vi "_word.table.Headers.vi"(7 "word.application":refnum<k7>, 8 "error in (no error)":errorcluster, 11 "table in":refnum<k7>) -> (0 "error out":errorcluster, 2 "table row contents":string[](array[string]), 3 "table out":refnum<k7>)   [LabVIEW 2018, in "WordReportGeneration.lvlib"]
uses:
  WordReportGeneration.lvlib
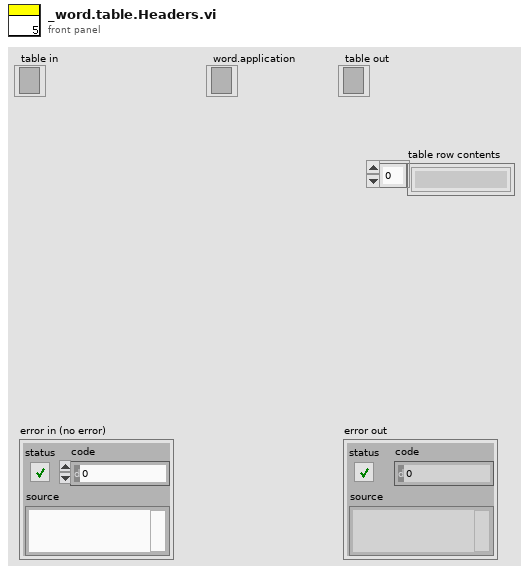
[diagram p1: front panel]
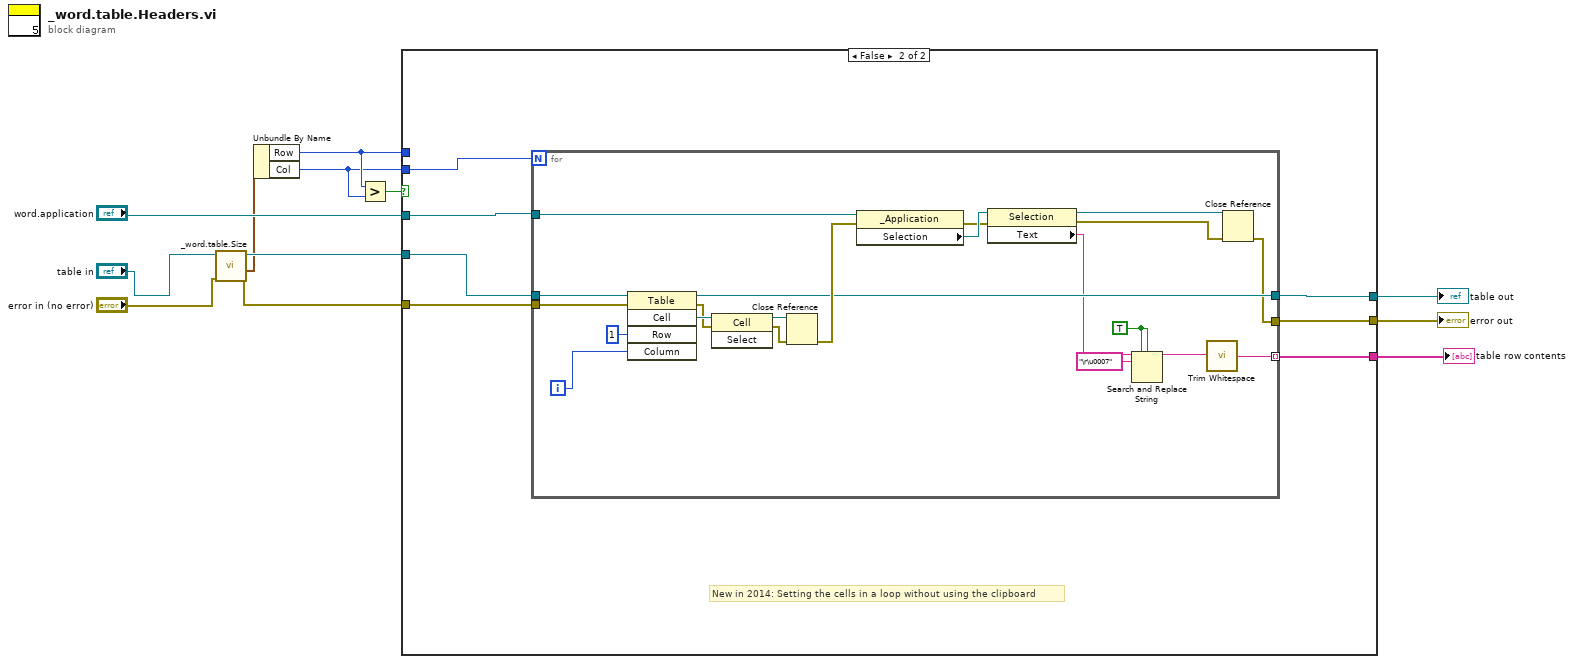
[diagram p0: block diagram]
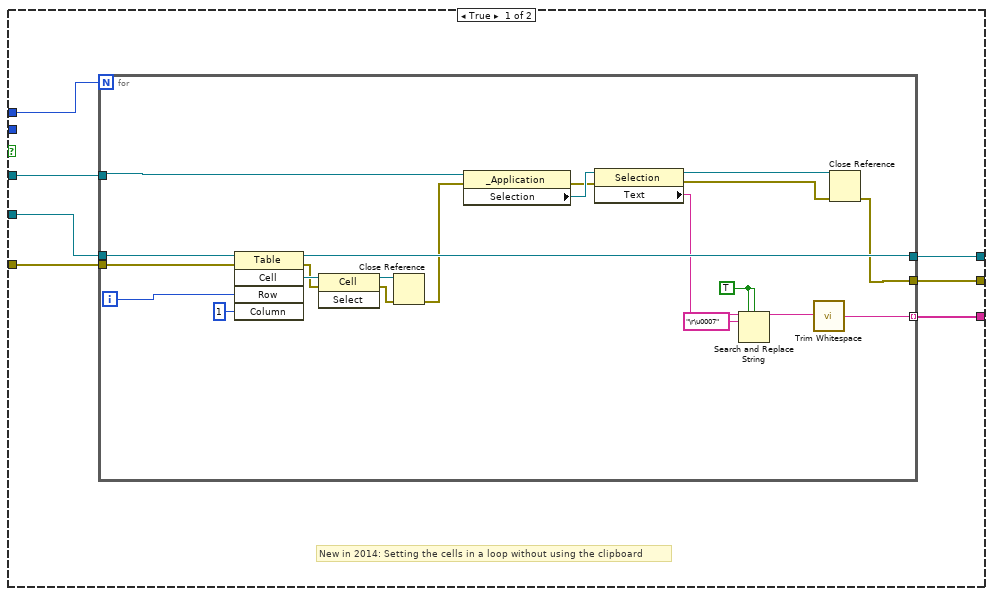
[diagram p2: hidden frame]
diagram:
  n1 = call "_word.table.Size.vi"("error in (no error)"="error in (no error)", "table Refnum in"="table in") -> ("error out"=w6:errorcluster, "Cluster"=w5:cluster{"Row":i32, "Col":i32}, "table Refnum out"=w8:refnum<k7>)  [unwired: 7 in]
  n2 = Unbundle By Name(w5) -> ("Row"=w4:i32, "Col"=w3:i32)
  n3 = Greater?(x=w4, y=w3) -> (0:w2:bool)
  n4 = case shown="False" w2 {
    tunnel: [w19 w47] -> w12
    tunnel: [w18 w46] -> w11
    tunnel: "word.application" -> [w17 w45]
    tunnel: w8 -> [w16 w44]
    tunnel: w6 -> [w15 w43]
    tunnel: [w13 w42] -> w1
    tunnel: w4 -> [w14 _]
    tunnel: w3 -> [_ w41]
    frame True {
      # "New in 2014: Setting the cells in a loop without using the clipboard"
      n5 = for {
        N: w14 -> [_]
        tunnel: [w40] -> w18
        tunnel: [w39] -> w19
        tunnel: w15 -> [w37]
        tunnel: w17 -> [w36]
        tunnel: w16 -> [w35]
        tunnel: [w34] -> w13 mode=indexing
        i -> [w38]
        w22 = TRUE ("ignore case? (F)")
        n6 = invoke class="Table" method="Cell"(reference=w35, error in=w37, "Row"=w38, "Column"=1) -> (reference out=w40:refnum<k7>, error out=w32:errorcluster, "Cell"=w33:refnum<k7>)  [unwired: 1 in, 2 out]
        n7 = invoke class="Cell" method="Select"(reference=w33, error in=w32) -> (reference out=w29:refnum<k7>, error out=w31:errorcluster)  [unwired: 1 in, 1 out]
        n8 = Close Reference(reference=w29, error in (no error)=w31) -> (error out=w30:errorcluster)
        n9 = property class="_Application"(reference=w36, error in=w30) -> (error out=w25:errorcluster, "Selection"=w26:refnum<k7>)  [unwired: 1 out]
        n10 = property class="Selection"(reference=w26, error in=w25) -> (reference out=w27:refnum<k7>, error out=w28:errorcluster, "Text"=w23:string)
        n11 = Search and Replace String(replace all?=w22, case sensitive?=w22, input string=w23, search string="\r\u0007") -> (result string=w24:string)  [unwired: 4 in, 3 out]
        n12 = call <vilib>:"Trim Whitespace.vi"("string"=w24) -> ("trimmed string"=w34:string)  [unwired: 1 in]
        n13 = Close Reference(reference=w27, error in (no error)=w28) -> (error out=w39:errorcluster)
      }
    }
    frame False {
      # "New in 2014: Setting the cells in a loop without using the clipboard"
      n14 = for {
        N: w41 -> [_]
        tunnel: [w63] -> w46
        tunnel: [w57] -> w47
        tunnel: w43 -> [w62]
        tunnel: w45 -> [w61]
        tunnel: w44 -> [w60]
        tunnel: [w53] -> w42 mode=indexing
        i -> [w54]
        w50 = TRUE ("ignore case? (F)")
        n15 = invoke class="Table" method="Cell"(reference=w60, error in=w62, "Row"=1, "Column"=w54) -> (reference out=w63:refnum<k7>, error out=w67:errorcluster, "Cell"=w68:refnum<k7>)  [unwired: 1 in, 2 out]
        n16 = invoke class="Cell" method="Select"(reference=w68, error in=w67) -> (reference out=w64:refnum<k7>, error out=w66:errorcluster)  [unwired: 1 in, 1 out]
        n17 = Close Reference(reference=w64, error in (no error)=w66) -> (error out=w65:errorcluster)
        n18 = property class="_Application"(reference=w61, error in=w65) -> (error out=w55:errorcluster, "Selection"=w56:refnum<k7>)  [unwired: 1 out]
        n19 = property class="Selection"(reference=w56, error in=w55) -> (reference out=w58:refnum<k7>, error out=w59:errorcluster, "Text"=w51:string)
        n20 = Search and Replace String(replace all?=w50, case sensitive?=w50, input string=w51, search string="\r\u0007") -> (result string=w52:string)  [unwired: 4 in, 3 out]
        n21 = call <vilib>:"Trim Whitespace.vi"("string"=w52) -> ("trimmed string"=w53:string)  [unwired: 1 in]
        n22 = Close Reference(reference=w58, error in (no error)=w59) -> (error out=w57:errorcluster)
      }
    }
  }
  "error out" <- w12
  "table out" <- w11
  "table row contents" <- w1
